vi "IOT抛网盘操作.vi"(11 "IOT DATA":string[](array[string])) -> ()   [LabVIEW 2017]
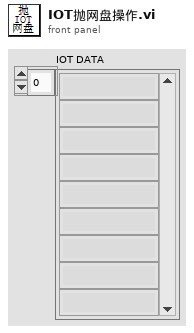
[diagram p1: front panel]
types:
  T1 = typedef "data格式选项.ctl" = enum16{"生成格式", "加载格式"}
  T2 = enum16{"open", "replace", "create", "open or create", "replace or create", "replace or create with confirmation"}
  T3 = typedef "表头集合.ctl" = cluster{"product信息":T4, "CT信息":T5, "ER信息":T6, "IOT信息":T7}
  T4 = typedef "product信息.ctl" = cluster{"product表头整合":string[], "量测部分表头":string[], "前侧贴合表头":string[], "后侧贴合表头":string[]}
  T5 = typedef "CT信息.ctl" = cluster{"CT表头整合":string[], "量测CT":string[], "动子1_2CT":string[], "动子3_4CT":string[]}
  T6 = typedef "ER信息.ctl" = cluster{"ER表头整合":string[]}
  T7 = typedef "IOT信息.ctl" = cluster{"IOT表头整合":string[]}
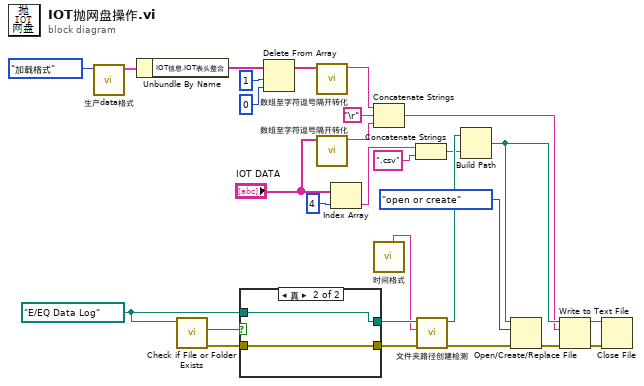
[diagram p0: block diagram]
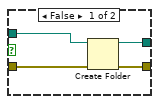
[diagram p2: hidden frame]
diagram:
  w27 = path "E:/EQ Data Log"
  n1 = call "生产data格式.vi"("data格式选项"=data格式选项."加载格式") -> ("表头格式"=w10:T3)  [unwired: 10 in]
  n2 = Unbundle By Name(w10) -> ("IOT信息.IOT表头整合"=w9:string[])
  n3 = call <vilib>:"Check if File or Folder Exists.vi"("path"=w27) -> ("error out"=w26:errorcluster, "file or folder exists?"=w28:bool)  [unwired: 8 in, 1 out]
  n4 = case shown="真" w28 {
    tunnel: w27 -> [w32 w34]
    tunnel: w26 -> [w31 w33]
    tunnel: [w30 w34] -> w25
    tunnel: [w29 w33] -> w23
    frame False {
      n5 = Create Folder(path (use dialog)=w32, error in=w31) -> (created path=w30:path, error out=w29:errorcluster)  [unwired: 1 in, 1 out]
    }
    frame True {
    }
  }
  n6 = Delete From Array(array=w9, length=1 ("长度"), index=0 ("长度")) -> (array with subset deleted=w5:string[])  [unwired: 1 out]
  n7 = call "数组至字符逗号隔开转化.vi"("数组data in"=w5) -> ("逗号隔开出"=w4:string)  [unwired: 10 in]
  n8 = call "数组至字符逗号隔开转化.vi"("数组data in"="IOT DATA") -> ("逗号隔开出"=w2:string)  [unwired: 10 in]
  n9 = Index Array(array="IOT DATA", index=4 ("索引")) -> (element=w18:string)
  n10 = Concatenate Strings(w4, "\r", w2) -> (w1:string)
  n11 = call "时间格式.vi"() -> ("Date"=w24:string)  [unwired: 7 in, 4 out]
  n12 = Concatenate Strings(w18, ".csv" ("字符串")) -> (w20:string)
  n13 = call "文件夹路径创建检测.vi"("error in (no error)"=w23, "文件夹名称"=w24, "基路径IN"=w25) -> ("error out"=w16:errorcluster, "路径OUT"=w22:path)  [unwired: 7 in]
  n14 = Build Path(base path=w22, name or relative path=w20) -> (appended path=w15:path)
  n15 = Open/Create/Replace File(file path (use dialog)=w15, error in=w16, operation (0:open)=T2."open or create" ("操作(0:open)")) -> (error out=w12:errorcluster)  [unwired: 3 in, 2 out]
  n16 = Write to Text File(file (use dialog)=w15, text=w1, error in=w12) -> (refnum out=w13:refnum<file>, error out=w14:errorcluster)  [unwired: 1 in, 1 out]
  n17 = Close File(refnum=w13, error in=w14) -> ()  [unwired: 2 out]
